vi "6 arduino lm35 Values only excel sheet.vi"() -> ()   [LabVIEW 2016]
uses:
  <vilib>/LabVIEW Interface for Arduino/Type Defs/Analog Pin.ctl
  <vilib>/LabVIEW Interface for Arduino/Type Defs/Board Type.ctl
  <vilib>/LabVIEW Interface for Arduino/Type Defs/Connection Type.ctl
  <vilib>/LabVIEW Interface for Arduino/LabVIEW Interface for Arduino.lvlib
panel:
  in  "stop":bool
  out "Waveform Chart":dbl(graph)
  in  "Baud Rate (115200)":u32=115200
  in  "Connection Type":T1
  in  "Board Type (Uno)":T2
  in  "file option":T3(ring)
  in  "file path (use dialog)":path=path "C:/Users/ASHWIN/Desktop/data/test1.txt"
  in  "access (0:read/write)":enum16{"read/write", "read-only", "write-only"}(ring)
  in  "Sekect COM port":refnum<visa-resource-name>="COM3"
  in  "Analog Pin":T4
  out "?":dbl(slide) scale=-50.0..150.0
  # "TEMPRATURE aNALYSIS AND  LOGGING"
  # "Developed by-\nAshlesh & Sudarshan"
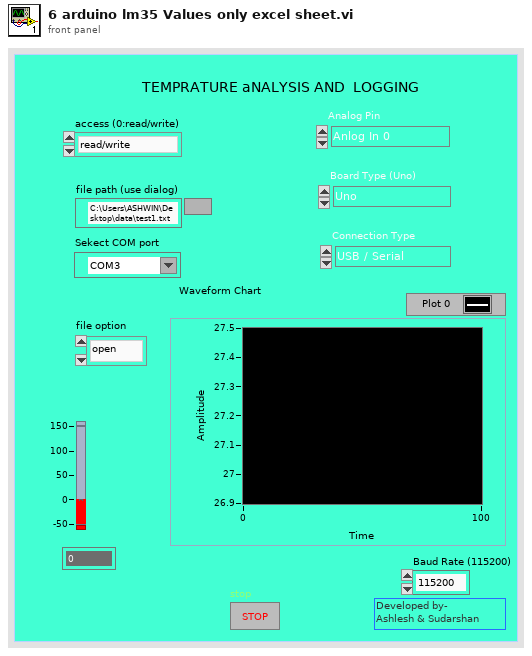
[diagram p1: front panel]
types:
  T1 = typedef "LabVIEW Interface for Arduino.lvlib/Connection Type.ctl" = enum8{"USB / Serial", "XBEE", "BlueSmirf (Bluetooth)"}
  T2 = typedef "LabVIEW Interface for Arduino.lvlib/Board Type.ctl" = enum16{"Uno", "Dimuelanove w/Atmega 328", "Mega 2560"}
  T3 = enum16{"open", "replace", "create", "open or create", "replace or create", "replace or create with confirmation"}
  T4 = typedef "LabVIEW Interface for Arduino.lvlib/Analog Pin.ctl" = enum8{"Anlog In 0", "Anlog In 1", "Anlog In 2", "Anlog In 3", "Anlog In 4", "Anlog In 5"}
  T5 = typedef "LabVIEW Interface for Arduino.lvlib/Arduino Resource.ctl" = cluster{"VISA resource":refnum<visa-resource-name>, "Board Type":T2, "Connection Type":enum8{"USB / Serial"}, "Bytes Per Packet (15)":u8}
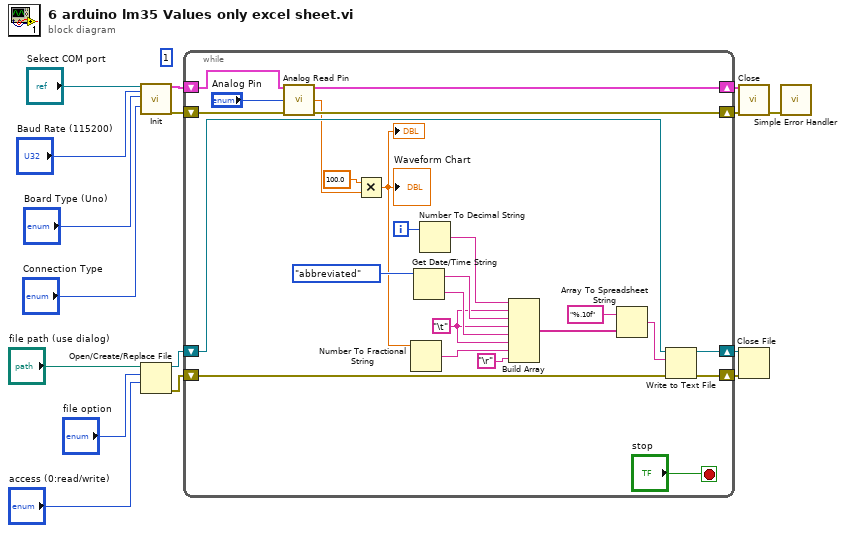
[diagram p0: block diagram]
diagram:
  (unwired) 1 ("Numeric")
  n1 = call <vilib>:"Init.vi"("VISA resource"="Sekect COM port", "Baud Rate (115200)"="Baud Rate (115200)", "Board Type (Uno)"="Board Type (Uno)", "Connection Type (USB/Serial)"="Connection Type") -> ("Arduino Resource"=w16:T5, "error out"=w13:errorcluster)  [unwired: 14 in]
  n2 = Open/Create/Replace File(file path (use dialog)="file path (use dialog)", operation (0:open)="file option", access (0:read/write)="access (0:read/write)") -> (refnum out=w5:refnum<file>, error out=w4:errorcluster)  [unwired: 1 in, 3 out]
  n3 = while {
    shift-right: [w40] -> w15
    shift-left: w16 -> [w38]
    shift-right: [w39] -> w14
    shift-left: w13 -> [w37]
    shift-right: [w31] -> w3
    shift-left: w5 -> [w33]
    shift-right: [w30] -> w2
    shift-left: w4 -> [w32]
    i -> [w26]
    stop <- "stop" stop-if-true
    w21 = "\t"
    n4 = call <vilib>:"Analog Read Pin.vi"("Arduino Resource"=w38, "Analog Input Pin (0)"="Analog Pin", "error in"=w37) -> ("Arduino Resource"=w40:T5, "Voltage"=w29:dbl, "error out"=w39:errorcluster)  [unwired: 10 in]
    n5 = Multiply(x=100.0, y=w29) -> (x*y=w18:dbl)
    "?" <- w18
    "Waveform Chart" <- w18
    n6 = Number To Fractional String(number=w18) -> (F-format string=w19:string)  [unwired: 3 in]
    n7 = Get Date/Time String(date format (0)=enum16{"short", "long", "abbreviated"}."abbreviated") -> (date string=w22:string, time string=w23:string)  [unwired: 2 in]
    n8 = Number To Decimal String(number=w26) -> (decimal integer string=w25:string)  [unwired: 1 in]
    n9 = Build Array(w25, w21, w22, w21, w23, w21, w19, "\r") -> (w34:string[])
    n10 = Array To Spreadsheet String(array=w34, 3:"%.10f") -> (spreadsheet string=w27:string)  [unwired: 1 out]
    n11 = Write to Text File(file (use dialog)=w33, text=w27, error in=w32) -> (refnum out=w31:refnum<file>, error out=w30:errorcluster)  [unwired: 1 in, 1 out]
  }
  n12 = call <vilib>:"Close.vi"("Arduino Resource"=w15, "error in"=w14) -> ("error out"=w12:errorcluster)  [unwired: 13 in]
  n13 = Close File(refnum=w3, error in=w2) -> ()  [unwired: 2 out]
  n14 = call <vilib>:"Simple Error Handler.vi"("error in (no error)"=w12) -> ()  [unwired: 4 in, 5 out]
